vi "Read BRAND SELECTED SIM.vi"(8 "error in (no error)":errorcluster, 11 "SIMULATED in":refnum<class "SIMULATED.lvclass">) -> (0 "error out":errorcluster, 2 "BRAND SELECTED":enum16{"NXP", "TI", "SIMULATED"}(ring), 3 "SIMULATED out":refnum<class "SIMULATED.lvclass">)   [LabVIEW 2019, in "SIMULATED.lvclass"]
uses:
  SIMULATED.lvclass
  SIMULATED.lvclass/SIMULATED.ctl
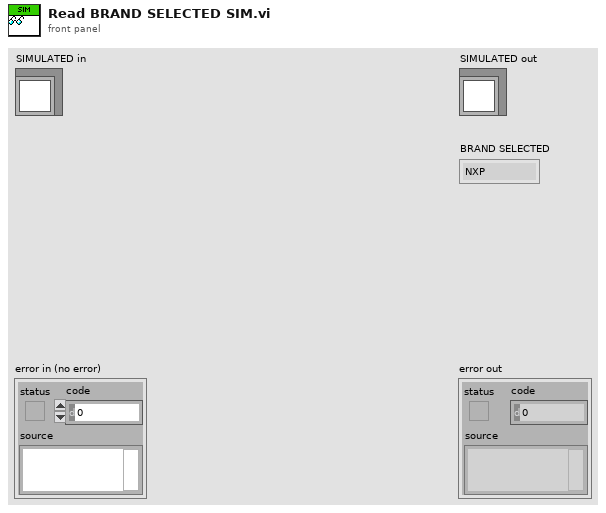
[diagram p1: front panel]
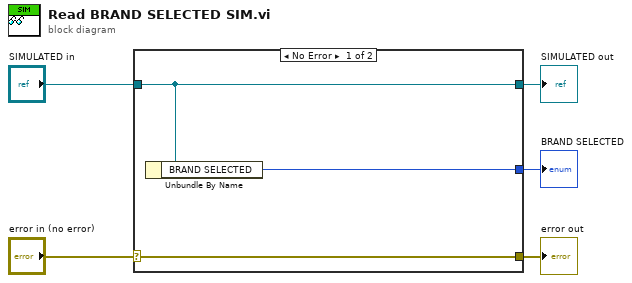
[diagram p0: block diagram]
diagram:
  n1 = case shown="No Error" "error in (no error)" {
    selector: "error in (no error)" -> [w8 w9]
    tunnel: [w8 w9] -> w4
    tunnel: [w7 w10] -> w2
    tunnel: "SIMULATED in" -> [w7 w10]
    tunnel: [w6 _] -> w1
    frame No Error {
      n2 = Unbundle By Name(w7) -> ("BRAND SELECTED"=w6:enum16{"NXP", "TI", "SIMULATED"})
    }
    frame Error {
    }
  }
  "error out" <- w4
  "SIMULATED out" <- w2
  "BRAND SELECTED" <- w1
